vi "__AWS Credentials Popup.vi"(8 "error in (no error)":errorcluster) -> (0 "error out":errorcluster, 2 "AWS Credentials":T1, 3 "Invalid Credentials":bool)   [LabVIEW 2011]
doc: "This is a pop-up dialog VI to request the user for the Access Key and Secret Key for Amazon S3."
uses:
  Typedefs/Access_Key_Type.ctl
  Typedefs/Secret_Key_Type.ctl
  vi.lib/National Instruments/LabVIEW Interface for Amazon S3/Typedefs/AMZ_S3_AWS Credentials.ctl
  vi.lib/National Instruments/LabVIEW Interface for Amazon S3/LV Interface for Amazon S3.lvlib
panel:
  in  "Cancel Button":bool
  in  "OK Button":bool
  in  "Secret Key":T2
  in  "Access Key":T3
  # "Please enter your AWS Credentials below!"
  # "To use this VI, you have to register first with Amazon\nto have an Amazon AWS account.\nIf you don't have an account yet, go to\nhttp://aws.amazon.com and Create an AWS account!"
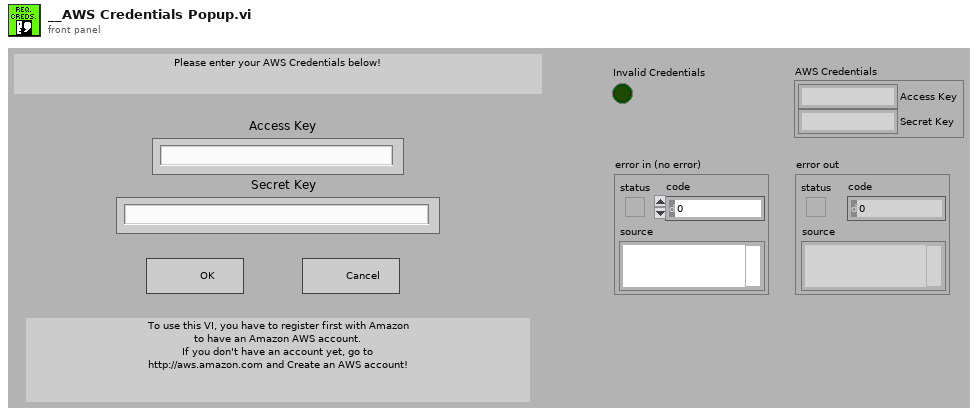
[diagram p1: front panel]
types:
  T1 = typedef "LV Interface for Amazon S3.lvlib/AMZ_S3_AWS Credentials.ctl" = cluster{"Access Key":string, "Secret Key":string}
  T2 = typedef "Secret_Key_Type.ctl" = string
  T3 = typedef "Access_Key_Type.ctl" = string
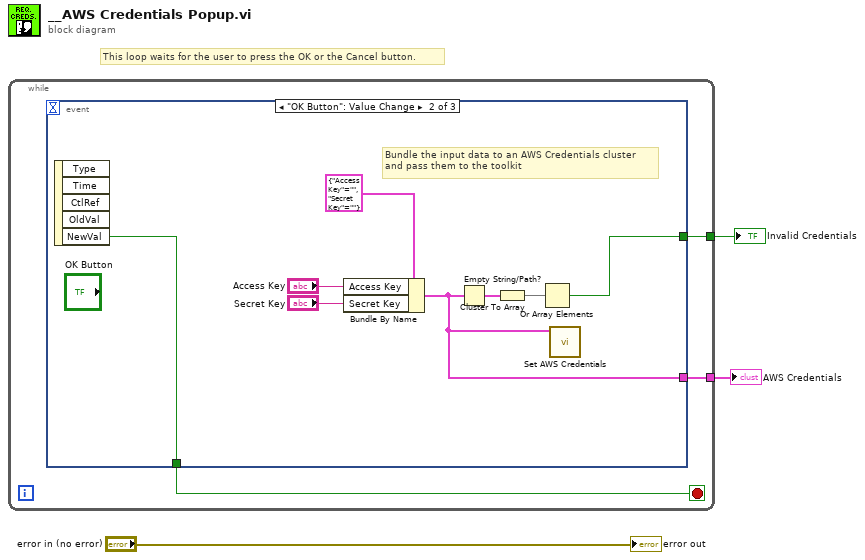
[diagram p0: block diagram]
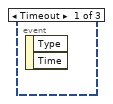
[diagram p2: hidden frame]
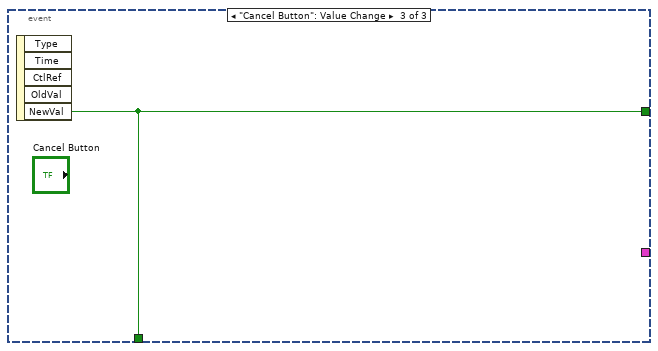
[diagram p3: hidden frame]
diagram:
  # "This loop waits for the user to press the OK or the Cancel button."
  n1 = while {
    tunnel: [w5] -> w3
    tunnel: [w4] -> w1
    stop <- w6 stop-if-true
    n2 = event shown="[1] \"OK Button\": Value Change" {
      selector: _ -> [_ _ _]
      dyn-events: _ -> [_ _ _]
      timeout: _ -> [_ _ _]
      tunnel: [_ w14 w15] -> w6
      tunnel: [_ w8 w15] -> w5
      tunnel: [_ w7 _] -> w4
      event Timeout {
        n3 = event-data() -> ()  [unwired: 1 in, 2 out]
      }
      event "OK Button": Value Change {
        # "Bundle the input data to an AWS Credentials cluster\nand pass them to the toolkit"
        n4 = event-data() -> ("NewVal"=w14:bool)  [unwired: 1 in, 4 out]
        n5 = Bundle By Name(cluster=T1 {"Access Key"="", "Secret Key"=""} ("AWS Credentials in"), "Access Key"="Access Key", "Secret Key"="Secret Key") -> (w7:T1)
        n6 = Empty String/Path?(string/path=w7) -> (empty?=w10:cluster{"Access Key":bool, "Secret Key":bool})
        n7 = Cluster To Array(cluster=w10) -> (array=w9:bool[])
        n8 = Or Array Elements(Boolean array=w9) -> (logical OR=w8:bool)
        n9 = call "Set AWS Credentials.vi"("AWS Credentials in"=w7) -> ()  [unwired: 10 in, 1 out]
      }
      event "Cancel Button": Value Change {
        n10 = event-data() -> ("NewVal"=w15:bool)  [unwired: 1 in, 4 out]
      }
    }
  }
  "Invalid Credentials" <- w3
  "AWS Credentials" <- w1
  "error out" <- "error in (no error)"
